vi "Read.vi"(8 "error in (no error)":errorcluster, 10 "LINX Resource in":T1, 11 "Address (0x27)":i8=39 format="%x") -> (0 "error out":errorcluster, 2 "LINX Resource out":T1, 3 "data":T7)   [LabVIEW 2015]
uses:
  <vilib>/MakerHub/LINX/Private/Type Defs/LINX Ref.ctl
  <vilib>/MakerHub/LINX/Private/Type Defs/Platform.ctl
  <vilib>/MakerHub/LINX/Private/Type Defs/Interface.ctl
  <vilib>/MakerHub/LINX/Private/Device/Type Defs/LINX Device Config.ctl
  <vilib>/MakerHub/LINX/Private/Device/Type Defs/TCP Config.ctl
  <vilib>/MakerHub/LINX/Private/Device/Type Defs/Channels.ctl
  <vilib>/MakerHub/LINX/Private/Local IO/LinxI2cWrite.vi
  <vilib>/MakerHub/LINX/Public/Utilities/Check Channel.vi
  <vilib>/MakerHub/LINX/Private/Utilties/Generate Error.vi
  <vilib>/MakerHub/LINX/LMH-LINX.lvlib
  <vilib>/MakerHub/LINX/Private/Device/Device.lvlib
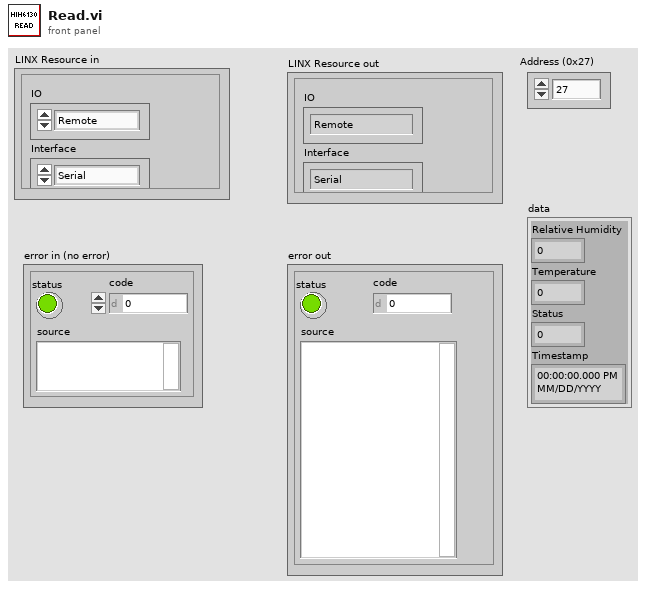
[diagram p1: front panel]
types:
  T1 = typedef "LMH-LINX.lvlib/LINX Ref.ctl" = cluster{"IO":T2, "Interface":T3, "LINX Device Config":T4}
  T2 = typedef "LMH-LINX.lvlib/Platform.ctl" = enum16{"Remote", "Local"}
  T3 = typedef "LMH-LINX.lvlib/Interface.ctl" = enum16{"Serial", "TCP"}
  T4 = typedef "LMH-LINX.lvlib/Device.lvlib/LINX Device Config.ctl" = cluster{"Interface":T3, "COM Port":refnum<visa-resource-name>, "TCP Configuration":T5, "Device Family":u8, "Device ID":u8, "Device Name":string, "TCP Ref":refnum<k5>, "Channels":T6}
  T5 = typedef "LMH-LINX.lvlib/Device.lvlib/TCP Config.ctl" = cluster{"IP Address":string, "Port":u16}
  T6 = typedef "LMH-LINX.lvlib/Channels.ctl" = cluster{"DI":u8[], "DO":u8[], "AI":u8[], "AO":u8[], "PWM":u8[], "QE":u8[], "UART":u8[], "I2C 2":u8[], "SPI":u8[], "CAN":u8[], "Servo":u8[], "AI Ref (V)":dbl, "AI Resolution (Bits)":u8, "AO Ref (V)":dbl, "AO Resolution (Bits)":u8}
  T7 = cluster{"Relative Humidity":dbl, "Temperature":dbl, "Status":i32, "Timestamp":timestamp}
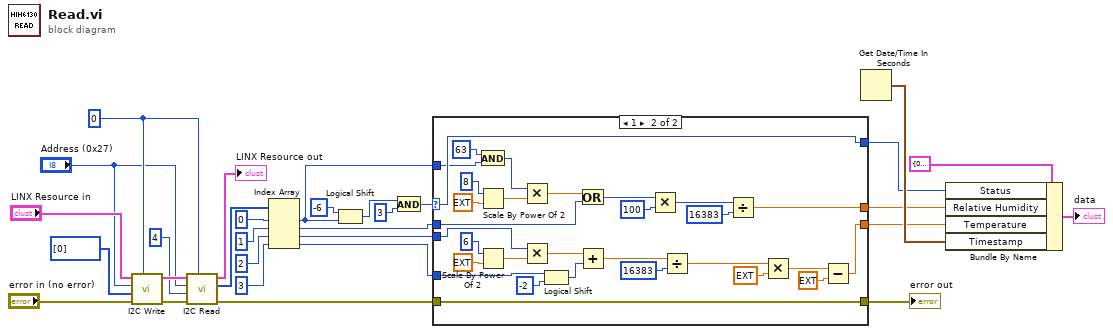
[diagram p0: block diagram]
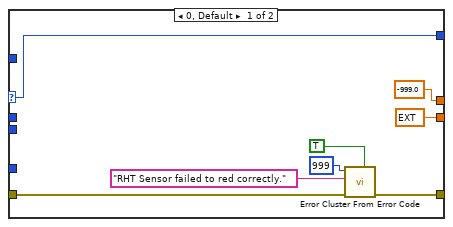
[diagram p2: hidden frame]
diagram:
  w27 = u8 0 ("I2C Channel")
  n1 = call <vilib>:"I2C Write.vi"("I2C Channel"=w27, "Error In"="error in (no error)", "Data"=u8[] [0], "I2C Slave Address (0)"="Address (0x27)", "LINX Resource"="LINX Resource in") -> ("Error Out"=w25:errorcluster, "LINX Resource"=w23:T1)  [unwired: 5 in]
  n2 = call <vilib>:"I2C Read.vi"("I2C Channel"=w27, "Error In"=w25, "Bytes To Read"=u8 4, "I2C Slave Address (0)"="Address (0x27)", "LINX Resource"=w23) -> ("Error Out"=w10:errorcluster, "Data"=w20:u8[], "LINX Resource"=→"LINX Resource out":T1)  [unwired: 4 in]
  n3 = Index Array(array=w20, index #1=0 ("index"), index #2=1 ("index"), index #3=2 ("index"), index #4=3 ("index")) -> (element #1=w1:u8, element #2=w8:u8, element #3=w7:u8, element #4=w6:u8)
  n4 = Logical Shift(y=i16 -6, x=w1) -> (x << y=w16:u8)
  n5 = And(x=w16, y=u8 3) -> (x .and. y?=w9:u8)
  n6 = case shown="1" w9 {
    selector: w9 -> [w33 w43]
    tunnel: w10 -> [w34 w68]
    tunnel: [w38 w68] -> w5
    tunnel: w8 -> [_ w42]
    tunnel: w7 -> [_ w41]
    tunnel: w6 -> [_ w40]
    tunnel: [ext -999.0 w45] -> w4
    tunnel: [-999.0 w44] -> w3
    tunnel: [w33 w43] -> w2
    tunnel: w1 -> [_ w39]
    frame 0, Default {
      n7 = call <vilib>:"Error Cluster From Error Code.vi"("is warning? (False)"=TRUE, "error in (no error)"=w34, "error message (\"\")"="RHT Sensor failed to red correctly." ("error message (\"\")"), "error code (0)"=999) -> ("error out"=w38:errorcluster)  [unwired: 5 in]
    }
    frame 1 {
      n8 = And(x=u8 63, y=w39) -> (x .and. y?=w62:u8)
      n9 = Scale By Power Of 2(n=i16 8 ("y"), x=ext 1.0) -> (x*2^n=w61:ext)
      n10 = Scale By Power Of 2(n=i16 6 ("y"), x=ext 1.0) -> (x*2^n=w55:ext)
      n11 = Multiply(x=w62, y=w61) -> (x*y=w58:ext)
      n12 = Multiply(x=w41, y=w55) -> (x*y=w54:ext)
      n13 = Logical Shift(y=w40, x=i8 -2) -> (x << y=w53:i8)
      n14 = Or(x=w58, y=w42) -> (x .or. y?=w66:i32)
      n15 = Add(x=w54, y=w53) -> (x+y=w51:ext)
      n16 = Multiply(x=w66, y=u8 100) -> (x*y=w64:i32)
      n17 = Divide(x=w51, y=u16 16383) -> (x/y=w49:ext)
      n18 = Divide(x=w64, y=u16 16383) -> (x/y=w44:dbl)
      n19 = Multiply(x=w49, y=ext 165.0) -> (x*y=w47:ext)
      n20 = Subtract(x=w47, y=ext 40.0) -> (x-y=w45:ext)
    }
  }
  "error out" <- w5
  n21 = Get Date/Time In Seconds() -> (seconds since 1Jan1904=w29:timestamp)
  n22 = Bundle By Name(cluster=T7 {"Relative Humidity"=0.0, "Temperature"=0.0, "Status"=0, "Timestamp"=timestamp(0 s since 1904-01-01)} ("input cluster"), "Status"=w2, "Relative Humidity"=w3, "Temperature"=w4, "Timestamp"=w29) -> (→"data":T7)
